vi "Expand Row Major Array.vi"(8 "Error in":errorcluster, 10 "Output Size (unreleased)":refnum<class "2D Array f32.lvclass">, 11 "1D Row Major In":refnum<class "1D Array binary.lvclass">) -> (0 "error out":errorcluster, 3 "2D Row Major Out":refnum<class "2D Array binary.lvclass">)   [LabVIEW 2020, in "G2CPU Line Profile.lvlib"]
uses:
  G2CPU Line Profile.lvlib
  <vilib>/Natan Biesmans/G2CPU GPU and CPU HPC Toolkit/G2CPU Libraries/Arrays/2DArray/binary/2D Array binary.lvclass
  C:/Program Files/National Instruments/LabVIEW 2025/vi.lib/Natan Biesmans/G2CPU GPU and CPU HPC Toolkit/G2CPU Libraries/Arrays/Array/Array Prototype.lvclass
  <vilib>/Natan Biesmans/G2CPU GPU and CPU HPC Toolkit/G2CPU Libraries/Arrays/1DArray/binary/1D Array binary.lvclass
  <vilib>/Natan Biesmans/G2CPU GPU and CPU HPC Toolkit/G2CPU Libraries/Arrays/2DArray/f32/2D Array f32.lvclass
  <vilib>/Natan Biesmans/G2CPU GPU and CPU HPC Toolkit/G2CPU Libraries/Arrays/2DArray/b8/2D Array s8.lvclass
  <vilib>/Natan Biesmans/G2CPU GPU and CPU HPC Toolkit/G2CPU Libraries/Arrays/Array/Array Prototype.lvclass/Array Prototype.ctl
  9f2e8118-353f-41e1-8f1c-d80ed56caf03.vi
  7379180f-d063-4741-98cc-50ebce035215.vi
  bdd9f843-be26-40f8-8bf2-00eaddede8bb.vi
  8947019b-5fa1-4a6f-92cf-d81b17d7e992.vi
  <vilib>/Natan Biesmans/G2CPU GPU and CPU HPC Toolkit/G2CPU Libraries/Arrays/Array/G2CPU Get Array Pointer Reference.vi
  <vilib>/Natan Biesmans/G2CPU GPU and CPU HPC Toolkit/G2CPU Libraries/Arrays/Array/G2CPU Set Array Pointer Reference.vi
  7379180f-d063-4741-98cc-50ebce035215.vi/cfed8f62-9c64-4dab-912e-5e7c21cb720b.vi
  <vilib>/Natan Biesmans/G2CPU GPU and CPU HPC Toolkit/G2CPU Libraries/Arrays/Array/G2CPU Get Array Pointer.vi
  bdd9f843-be26-40f8-8bf2-00eaddede8bb.vi/5793b77b-c002-4ebf-9075-685617c95341.vi
  bdd9f843-be26-40f8-8bf2-00eaddede8bb.vi/2ed3ef86-c00d-4d71-b84c-20267a6dfcf9.vi
  7379180f-d063-4741-98cc-50ebce035215.vi/cfed8f62-9c64-4dab-912e-5e7c21cb720b.vi/77c7badc-ed81-4514-99c1-20d37f4e5ecc.vi
  7379180f-d063-4741-98cc-50ebce035215.vi/cfed8f62-9c64-4dab-912e-5e7c21cb720b.vi/eb76fa01-6782-47b4-b34f-9eb474c9cc78.vi
  <vilib>/Natan Biesmans/G2CPU GPU and CPU HPC Toolkit/ArrayFire Driver/VIs/Run as Multi Device.vi
  bdd9f843-be26-40f8-8bf2-00eaddede8bb.vi/5793b77b-c002-4ebf-9075-685617c95341.vi/3e802c67-fb96-46a3-ae13-4994a8508b4f.vi
  bdd9f843-be26-40f8-8bf2-00eaddede8bb.vi/5793b77b-c002-4ebf-9075-685617c95341.vi/5a50fc67-79e7-4972-80c2-92243cd53dd4.vi
  bdd9f843-be26-40f8-8bf2-00eaddede8bb.vi/2ed3ef86-c00d-4d71-b84c-20267a6dfcf9.vi/730f6c57-5c0b-4ee9-b61e-75067b25222b.vi
  bdd9f843-be26-40f8-8bf2-00eaddede8bb.vi/2ed3ef86-c00d-4d71-b84c-20267a6dfcf9.vi/096b8799-7810-404e-baca-ba9279cec4bd.vi
  bdd9f843-be26-40f8-8bf2-00eaddede8bb.vi/2ed3ef86-c00d-4d71-b84c-20267a6dfcf9.vi/0f1a5a47-bcc5-4796-ac31-8dfcfbc0d7d1.vi
  bdd9f843-be26-40f8-8bf2-00eaddede8bb.vi/2ed3ef86-c00d-4d71-b84c-20267a6dfcf9.vi/89f12e17-3330-4b72-ad8f-8dd636660732.vi
  <vilib>/Natan Biesmans/G2CPU GPU and CPU HPC Toolkit/ArrayFire Driver/VIs/iszero.vi
  <vilib>/Natan Biesmans/G2CPU GPU and CPU HPC Toolkit/ArrayFire Driver/VIs/sub.vi
  <vilib>/Natan Biesmans/G2CPU GPU and CPU HPC Toolkit/ArrayFire Driver/VIs/release array.vi
  <vilib>/Natan Biesmans/G2CPU GPU and CPU HPC Toolkit/ArrayFire Driver/subvi/Error Converter (ErrCode or Status).vi
  <vilib>/Natan Biesmans/G2CPU GPU and CPU HPC Toolkit/ArrayFire Driver/VIs/cast.vi
  <vilib>/Natan Biesmans/G2CPU GPU and CPU HPC Toolkit/ArrayFire Driver/VIs/add.vi
  <vilib>/Natan Biesmans/G2CPU GPU and CPU HPC Toolkit/G2CPU Libraries/Arrays/Array/G2CPU Set Array Pointer.vi
  <vilib>/Natan Biesmans/G2CPU GPU and CPU HPC Toolkit/G2CPU Libraries/Arrays/SubVI/is 2D.vi
  <vilib>/Natan Biesmans/G2CPU GPU and CPU HPC Toolkit/G2CPU Libraries/Arrays/Array/G2CPU Release Array.vi
  <vilib>/Natan Biesmans/G2CPU GPU and CPU HPC Toolkit/G2CPU Libraries/Arrays/1DArray/b8/1D Array s8.lvclass
  <vilib>/Natan Biesmans/G2CPU GPU and CPU HPC Toolkit/G2CPU Libraries/Arrays/2DArray/2D Array Prototype.lvclass
  <vilib>/Natan Biesmans/G2CPU GPU and CPU HPC Toolkit/G2CPU Libraries/Arrays/Array/Array Prototype.lvclass
  <vilib>/Natan Biesmans/G2CPU GPU and CPU HPC Toolkit/G2CPU Libraries/Arrays/DataTypes/I8/s8.lvclass
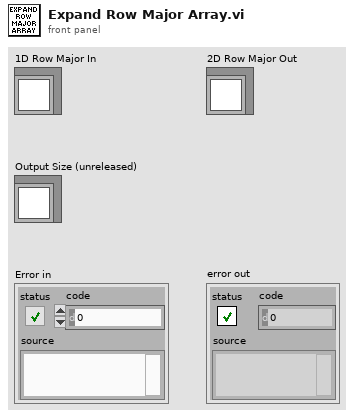
[diagram p1: front panel]
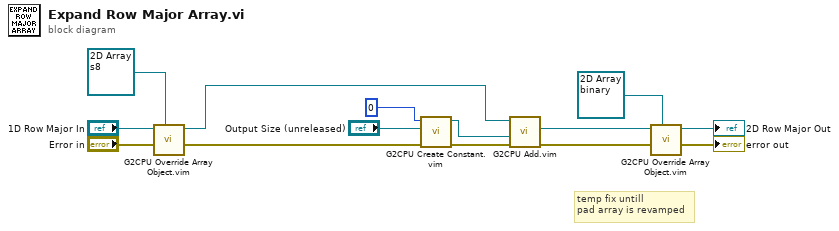
[diagram p0: block diagram]
diagram:
  # "temp fix untill \npad array is revamped"
  n1 = call "G2CPU Override Array Object.vim"("New Array Type"=refnum<class "2D Array s8.lvclass"> refnum ("Output Size (Mapped) 2"), "error in (no error)"="Error in", "To Override Array"="1D Row Major In") -> ("error out"=w8:errorcluster, "Overriden Array (inplace)"=w5:refnum<class "2D Array s8.lvclass">)  [unwired: 7 in]
  n2 = call "G2CPU Create Constant.vim"("error in (no error)"=w8, "Size"="Output Size (unreleased)", "val"=i8 0) -> ("error out"=w3:errorcluster, "object out"=w4:refnum<class "2D Array s8.lvclass">)  [unwired: 7 in]
  n3 = call "G2CPU Add.vim"("error in (no error)"=w3, "Array rhs"=w4, "Array lhs"=w5) -> ("error out"=w1:errorcluster, "Array Result"=w2:refnum<class "2D Array s8.lvclass">)  [unwired: 7 in]
  n4 = call "G2CPU Override Array Object.vim"("New Array Type"=refnum<class "2D Array binary.lvclass"> refnum ("G2CPU Arrays.lvlib:2D Array binary.lvclass"), "error in (no error)"=w1, "To Override Array"=w2) -> ("error out"=→"error out":errorcluster, "Overriden Array (inplace)"=→"2D Row Major Out":refnum<class "2D Array binary.lvclass">)  [unwired: 7 in]
